vi "RunningAverage.vi"(9 "New Image":dbl[][](array[numeric]), 10 "# of Averages for the Old Image":u32=1, 11 "Old Image":dbl[][](array[numeric])) -> (3 "Averaged Image":dbl[][](array[numeric]))   [LabVIEW 2018]
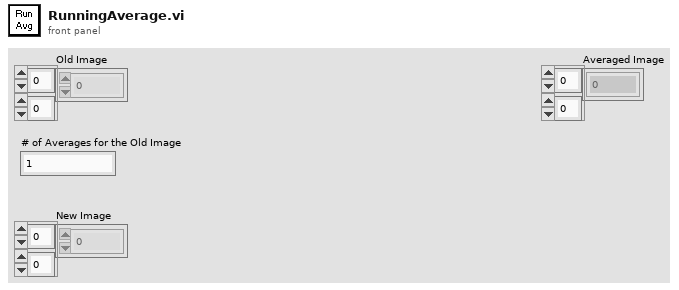
[diagram p1: front panel]
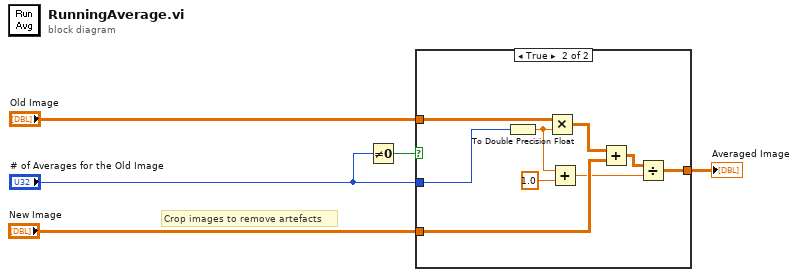
[diagram p0: block diagram]
diagram:
  # "Crop images to remove artefacts"
  n1 = Not Equal To 0?(x="# of Averages for the Old Image") -> (x != 0?=w2:bool)
  n2 = case shown="True" w2 {
    tunnel: "Old Image" -> [_ w15]
    tunnel: "# of Averages for the Old Image" -> [_ w14]
    tunnel: "New Image" -> [w6 w12]
    tunnel: [w6 w7] -> w3
    frame False {
    }
    frame True {
      n3 = To Double Precision Float(number=w14) -> (double precision float=w10:dbl)
      n4 = Multiply(x=w15, y=w10) -> (x*y=w13:dbl[][])
      n5 = Add(x=w10, y=1.0) -> (x+y=w8:dbl)
      n6 = Add(x=w13, y=w12) -> (x+y=w11:dbl[][])
      n7 = Divide(x=w11, y=w8) -> (x/y=w7:dbl[][])
    }
  }
  "Averaged Image" <- w3
